vi "test Random Data Plugin Run.vi"(8 "error in (no error)":errorcluster, 11 "TestCase in":refnum<class "Data Engine Unit Tests.lvclass">) -> (0 "error out":errorcluster, 3 "TestCase out":refnum<class "Data Engine Unit Tests.lvclass">)   [LabVIEW 2017, in "Data Engine Unit Tests.lvclass"]
uses:
  Data Engine Unit Tests.lvclass
  Source/Random Data Plugin/Random Data Plugin.lvclass
  D:/xtra/vi/Data Engine/Data Plugin/Data Plugin.lvclass
  <vilib>/addons/_JKI Toolkits/VI Tester/TestCase.llb/TestCase.lvclass
  C:/Program Files/National Instruments/LabVIEW 2017/vi.lib/addons/_JKI Toolkits/VI Tester/TestCase.llb/TestCase.lvclass
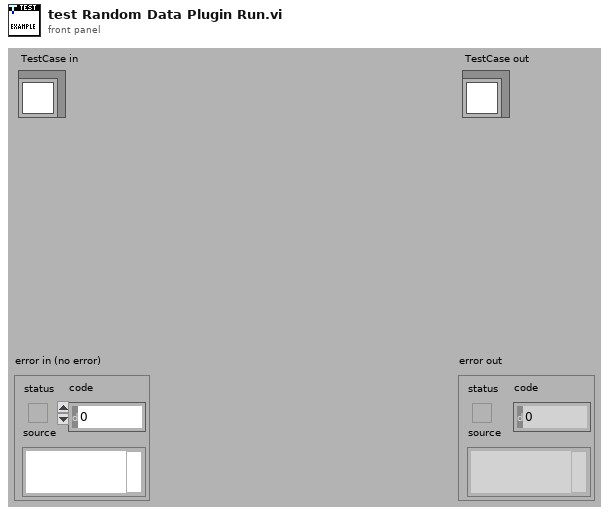
[diagram p1: front panel]
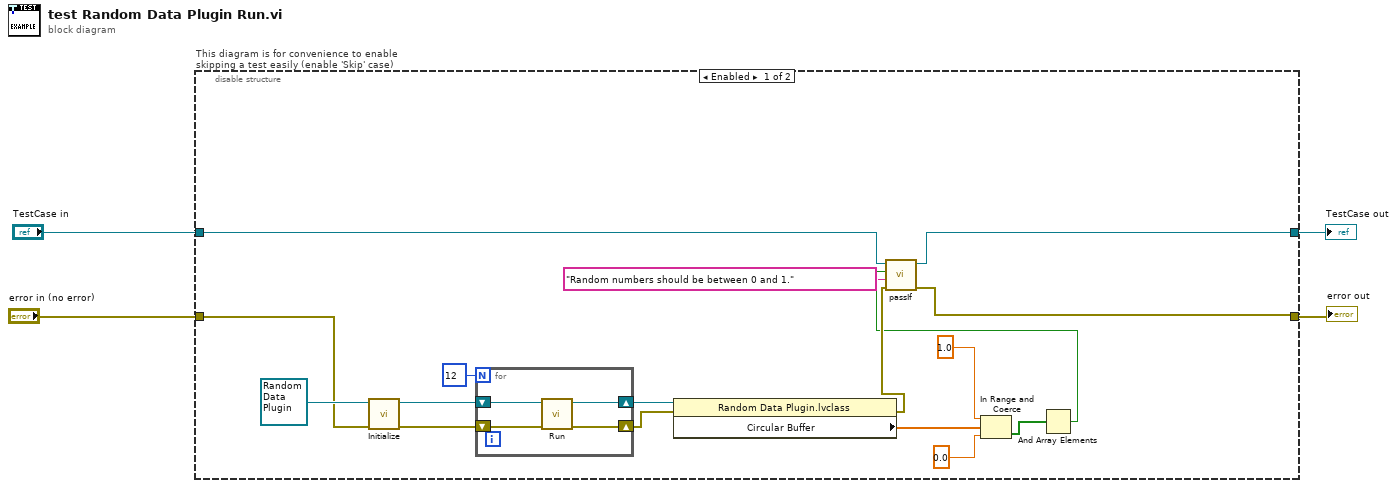
[diagram p0: block diagram]
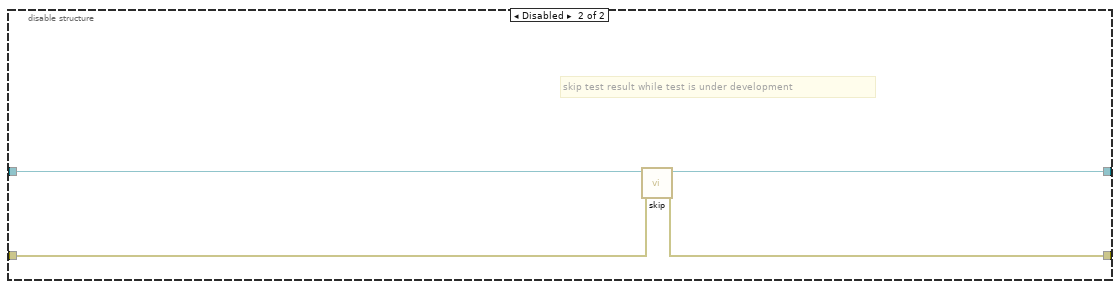
[diagram p2: hidden frame]
diagram:
  n1 = disable-structure "This diagram is for convenience to enable skipping a test easily (enable 'Skip' case)" shown="Enabled" {
    disable-tunnel: "TestCase in" -> [w21 w29]
    disable-tunnel: [w20 w27] -> w1
    disable-tunnel: [w19 w28] -> w3
    disable-tunnel: "error in (no error)" -> [w14 w26]
    frame Enabled {
      n2 = call-dynamic "Initialize.vi"("error in (no error)"=w14, "Data Plugin in"=refnum<class "Random Data Plugin.lvclass"> refnum ("Data Engine.lvlib:Random Data Plugin.lvclass")) -> ("error out"=w15:errorcluster, "Data Plugin out"=w16:refnum<class "Random Data Plugin.lvclass">)  [unwired: 8 in]
      n3 = for {
        N: 12 -> [_]
        shift-right: [w24] -> w13
        shift-left: w16 -> [w25]
        shift-right: [w22] -> w12
        shift-left: w15 -> [w23]
        n4 = call-dynamic "Run.vi"("error in (no error)"=w23, "Data Plugin in"=w25) -> ("error out"=w22:errorcluster, "Data Plugin out"=w24:refnum<class "Random Data Plugin.lvclass">)  [unwired: 8 in]
      }
      n5 = property class="Random Data Plugin.lvclass"(reference=w13, error in=w12) -> (error out=w11:errorcluster, "Circular Buffer"=w10:dbl[])  [unwired: 1 out]
      n6 = In Range and Coerce(upper limit=1.0, x=w10, lower limit=0.0) -> (In Range?=w7:bool[])  [unwired: 1 out]
      n7 = And Array Elements(Boolean array=w7) -> (logical AND=w6:bool)
      n8 = call-dynamic "passIf.vi"("error in (no error)"=w11, "message (\"\")"="Random numbers should be between 0 and 1." ("message (\"\")"), "pass"=w6, "TestCase in"=w21) -> ("error out"=w19:errorcluster, "TestCase out"=w20:refnum<class "Data Engine Unit Tests.lvclass">)  [unwired: 6 in]
    }
    frame Disabled {
      # "skip test result while test is under development"
      n9 = call <vilib>:"skip.vi"("error in (no error)"=w26, "TestCase in"=w29) -> ("error out"=w28:errorcluster, "TestCase out"=w27:refnum<class "Data Engine Unit Tests.lvclass">)  [unwired: 8 in]
    }
  }
  "error out" <- w3
  "TestCase out" <- w1
